vi "Global_var.vi"() -> ()   [LabVIEW 2020]
panel:
  in  "bitrate":u32=512000
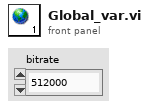
[diagram p1: front panel]
diagram:
